vi "ROTPEN Swing-Up_for_student.vi"() -> ()   [LabVIEW 2018]
uses:
  <vilib>/Simulation/Scripting/Companion Diagram/SimConfigNode/SimParams.ctl
  <vilib>/Simulation/Scripting/Companion Diagram/SimConfigNode/_simSolvers.ctl
  <vilib>/Simulation/Implementation/Shared/SIMSCR Execution Mode.ctl
  <vilib>/Platform/TimedLoop/XDataNode/timing_clust.ctl
  <vilib>/Platform/TimedLoop/XDataNode/nitl_modes.ctl
  <vilib>/Platform/TimedLoop/XDataNode/wakeup.ctl
  <vilib>/Simulation/Param Hierarchy/Typedefs/SIMPH Param Control Actions.ctl
  <vilib>/Simulation/Scripting/Editor Utilities/SIM subVI tag data.ctl
  <vilib>/Simulation/Scripting/Editor Utilities/SIM subVI execution type.ctl
  <vilib>/Simulation/Implementation/Shared/NILVSim_ParamChanged.vi
  <vilib>/Simulation/Implementation/Shared/NILVSim_FinishedLate.vi
  <vilib>/Simulation/Implementation/Shared/NILVSIM_BeginStep.vi
  <vilib>/Simulation/DataSources/Implementation/NILVSim Signal Generator.llb/SIM Signal Generator (scalar).vi
  <vilib>/Simulation/SignalArithmetic/Implementation/NILVSim Gain.llb/SIM Gain (scalar).vi
  <vilib>/Simulation/Utility/Implementation/SIM Halt.vi
  <vilib>/Simulation/ContinuousLinear/Implementation/NILVSim Transfer Function Direct.llb/SIM Transfer Function Direct (SISO).vi
  <vilib>/Simulation/Nonlinear/Implementation/NILVSim Saturation.llb/SIM Saturation (scalar).vi
  <vilib>/Simulation/SignalArithmetic/Implementation/NILVSim Gain.llb/SIM Gain (vector,MatrixGain).vi
  <vilib>/Simulation/Implementation/Shared/SIM Fire Discrete SubVI.vi
  <vilib>/Simulation/Implementation/Shared/NILVSim_Manager.vi
  <vilib>/Utility/error.llb/Clear Errors.vi
  <vilib>/Simulation/Implementation/Shared/NILVSim_FinalizeModel.vi
  <vilib>/Simulation/Implementation/Shared/SIM Fire Discrete SubVI (Core).vi
  <vilib>/Simulation/Implementation/Shared/SIM Unbundle Sim Info.vi
  <vilib>/Simulation/Implementation/Shared/SIMSH Read Queue.vi
  <vilib>/Simulation/Implementation/Shared/NILVSim_Initialize.vi
  <vilib>/Simulation/Utility/Implementation/NILVSim Get Time and IsAcceptedStep.vi
  <vilib>/imath/engines/lvmath2/RunTimeEngine/NodeEndStatement/NIMS_NodeEndStatement_Output.vi
  <instcachedir>/0/NIMS_NodeEndStatement_Output_53EC0D466D134D7ABD903AC30B43404B.lvgen/NIMS_NodeEndStatement_Output_53EC0D466D134D7ABD903AC30B43404B_001.vi
  <vilib>/imath/engines/lvmath2/RunTimeEngine/ErrorHandling/NIMS_Finalize Error.vi
  <vilib>/Simulation/Implementation/Shared/NILVSim_GetModelError.vi
  <vilib>/Simulation/Implementation/Shared/SIM Bundle Sim Info.vi
  <vilib>/Simulation/Scripting/Companion Diagram/SimConfigNode/SimDog.xnode
  <vilib>/Quanser/Rapid Control Prototyping Toolkit/hardware/HIL Immediate IO/_TypeSpecific/CL HIL Write Analog (Scalar).vi
  <vilib>/Quanser/Rapid Control Prototyping Toolkit/hardware/HIL Immediate IO/CL HIL Write.vi
  <vilib>/Quanser/Rapid Control Prototyping Toolkit/hardware/HIL Immediate IO/_TypeSpecific/CL HIL Read Encoder (Vector).vi
  <vilib>/Quanser/Rapid Control Prototyping Toolkit/hardware/HIL Immediate IO/CL HIL Read.vi
  <vilib>/Platform/TimedLoop/XDataNode/XDataNode.xnode
  <vilib>/Simulation/Implementation/XNodeFramework/SimXNode/SimX.xnode
  <vilib>/Platform/TimedLoop/XDataNode/XDNodeRunTimeDep.lvlib
  <vilib>/Simulation/Implementation/Shared/NI_SIM_Implementation.lvlib
panel:
  in  "kp":dbl=5.0
  out "out":dbl=1.7286661490025967
  out "Motor Voltage (V)  2":dbl(graph)=19.319735862133093
  in  "Enable control":bool
  in  "Er (J)":dbl=0.42
  in  "mu":dbl=46.0
  in  "u_max (m/s^2)":dbl=70.0
  in  "Pendulum Model Parameters":T1={"Mp (kg)"=0.127, "Mr (kg)"=0.257, "Lr (m)"=0.2159, "Lp (m)"=0.3365, "Jr (kg.m^2)"=0.001, "Dr (N.m.s/rad)"=0.0024, "Jp (kg.m^2)"=0.0012, "Dp (N.m.s/rad)"=0.0024, "g (m/s^2)"=9.81} {"Mr (kg)" min=0.0 format="%_3f"; "g (m/s^2)" min=0.0 format="%_3g"; "Lr (m)" min=0.0 format="%_3g"; "Dr (N.m.s/rad)" min=0.0 format="%_3g"; "Jr (kg.m^2)" min=0.0 format="%_3g"; "Dp (N.m.s/rad)" min=0.0 format="%_3g"; "Jp (kg.m^2)" min=0.0 format="%_3g"; "Lp (m)" min=0.0 format="%_3g"; "Mp (kg)" min=0.0 format="%_3f"}
  in  "SRV02 Model Parameters":T2={"Rm (ohm)"=2.6, "km (V-s/rad)"=0.00767, "kt (N-m/A)"=0.00767, "Jm (kg-m^2)"=4.6000000000000004e-07, "Dm (N-m-s/rad)"=0.0, "Jg (kg.m^2)"=5.28e-05, "JL (kg.m^2)"=5e-05, "DL (N-m-s/rad)"=0.015, "Kg"=70} {"Jg (kg.m^2)" min=0.0 format="%_3g"; "Dm (N-m-s/rad)" min=0.0 format="%_3g"; "Kg" min=0; "DL (N-m-s/rad)" min=0.0 format="%_3g"; "JL (kg.m^2)" min=0.0 format="%_3g"; "Jm (kg-m^2)" min=0.0 format="%_3g"; "kt (N-m/A)" min=0.0 format="%_3g"; "km (V-s/rad)" min=0.0 format="%_3g"; "Rm (ohm)" min=0.0 format="%_3f"}
  out "E (J)":dbl=5.742127541452646e-06
  in  "stop":bool
  in  "Feedback Gain":dbl[][](array[numeric])=[[-5.3, 28.3, -2.8, 3.2]]
  out "Motor Voltage (V)":dbl(graph)
  out "Rotary Arm Position (deg)":cluster{"output":dbl, "output":dbl}(graph)={"output"=0.0, "output"=-0.878909632226957}
  out "Pendulum Angle (deg)":dbl(graph)=179.73701979041272
  in  "Frequency (Hz)":dbl(slide)=0.2 min=0.0 max=0.5 step=0.05 scale=0.0..0.5 scale format="%#_3f"
  in  "Amplitude (deg)":dbl(slide) min=0.0 max=40.0 step=5.0 scale=0.0..40.0
  # "Rotary Arm Reference Signal"
  # "Swing-Up Parameters"
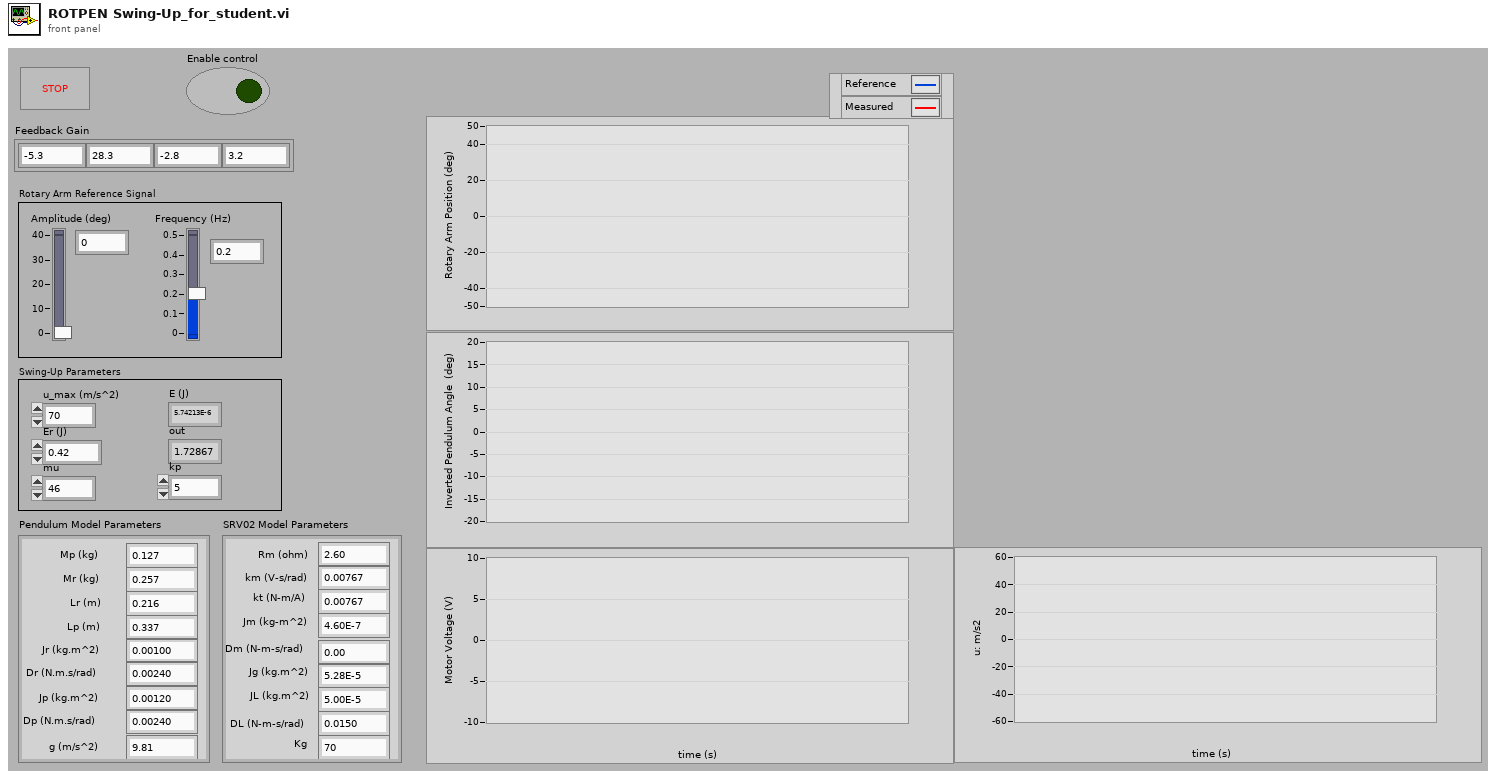
[diagram p1: front panel]
types:
  T1 = cluster{"Mp (kg)":dbl, "Mr (kg)":dbl, "Lr (m)":dbl, "Lp (m)":dbl, "Jr (kg.m^2)":dbl, "Dr (N.m.s/rad)":dbl, "Jp (kg.m^2)":dbl, "Dp (N.m.s/rad)":dbl, "g (m/s^2)":dbl}
  T2 = cluster{"Rm (ohm)":dbl, "km (V-s/rad)":dbl, "kt (N-m/A)":dbl, "Jm (kg-m^2)":dbl, "Dm (N-m-s/rad)":dbl, "Jg (kg.m^2)":dbl, "JL (kg.m^2)":dbl, "DL (N-m-s/rad)":dbl, "Kg":i16}
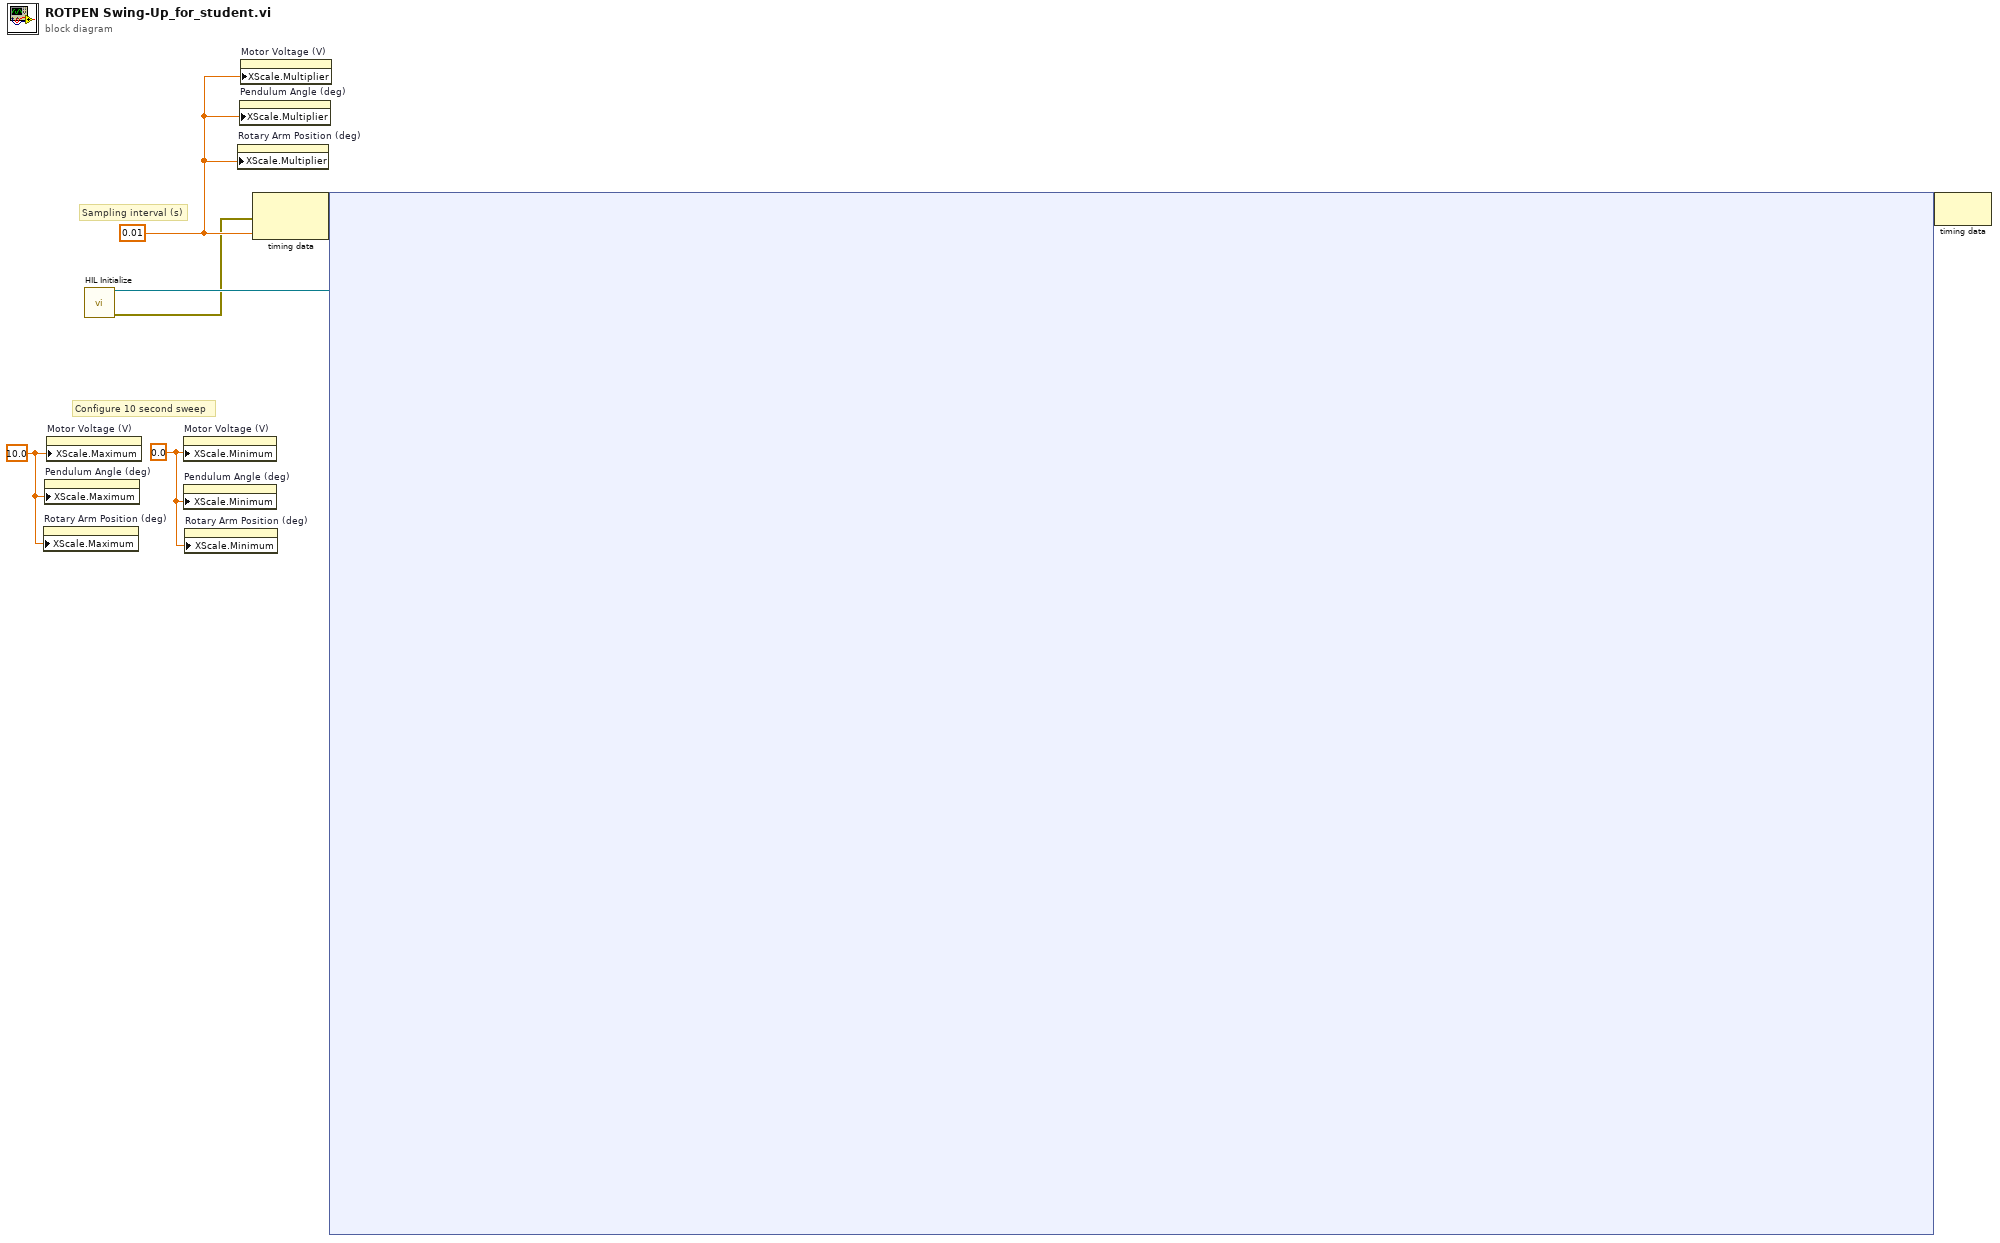
[diagram p0: block diagram]
diagram:
  w2 = 0.0 ("X Scale.Range:Maximum")
  w3 = 10.0 ("X Scale.Range:Maximum")
  w4 = 0.01 ("Step Size (s)")
  # "Configure 10 second sweep"
  # "Sampling interval (s)"
  n1 = property on="Rotary Arm Position (deg)" class="WFChart (strict)"("XScale.Maximum"=w3) -> ()  [unwired: 2 in, 2 out]
  n2 = property on="Pendulum Angle (deg)" class="WFChart (strict)"("XScale.Maximum"=w3) -> ()  [unwired: 2 in, 2 out]
  n3 = property on="Motor Voltage (V)" class="WFChart (strict)"("XScale.Maximum"=w3) -> ()  [unwired: 2 in, 2 out]
  n4 = call "HIL Initialize"() -> ("board out"=w5:refnum<class "HIL Board.lvclass">, "error out"=w1:errorcluster)  [unwired: 14 in]
  n5 = property on="Motor Voltage (V)" class="WFChart (strict)"("XScale.Minimum"=w2) -> ()  [unwired: 2 in, 2 out]
  n6 = property on="Pendulum Angle (deg)" class="WFChart (strict)"("XScale.Minimum"=w2) -> ()  [unwired: 2 in, 2 out]
  n7 = property on="Rotary Arm Position (deg)" class="WFChart (strict)"("XScale.Minimum"=w2) -> ()  [unwired: 2 in, 2 out]
  n8 = property on="Rotary Arm Position (deg)" class="WFChart (strict)"("XScale.Multiplier"=w4) -> ()  [unwired: 2 in, 2 out]
  n9 = property on="Pendulum Angle (deg)" class="WFChart (strict)"("XScale.Multiplier"=w4) -> ()  [unwired: 2 in, 2 out]
  n10 = property on="Motor Voltage (V)" class="WFChart (strict)"("XScale.Multiplier"=w4) -> ()  [unwired: 2 in, 2 out]
  n11 = node-c288(w1, w4) -> (w7:variant)
  n12 = node-c254 ("Control & Simulation Loop")(w7, w5) -> (w6:variant)
  n13 = node-c288(w6) -> ()  [unwired: 1 out]
